vi "Initialize.vi"(7 "Channel Name":string="Setpoint.ch%d.SP", 8 "error in":errorcluster, 9 "Number of Channels":u32=1, 10 "Instance Name":string, 11 "Output Enable in":refnum<class "Output Enable.lvclass">) -> (0 "error out":errorcluster, 3 "Output Enable out":refnum<class "Output Enable.lvclass">)   [LabVIEW 2023, in "Output Enable.lvclass"]
uses:
  Output Enable.lvclass
  Output Enable.lvclass/Output Enable.ctl
  <vilib>/ADAS Replay HIL/Channels/Tag Wrapper/Tag Wrapper.lvlib
  Utilities/Utilities.lvlib
  <vilib>/ADAS Replay HIL/Channels/Tag Wrapper/Polymorphic/Set Default Value (Boolean).vi
  <vilib>/ADAS Replay HIL/Channels/Tag Wrapper/Polymorphic/Open Consumer Tag (Boolean).vi
  <vilib>/ADAS Replay HIL/Channels/Tag Wrapper/Polymorphic/Open Producer Tag (I32).vi
  <vilib>/ADAS Replay HIL/Channels/Tag Wrapper/Polymorphic/Set Default Value (I32).vi
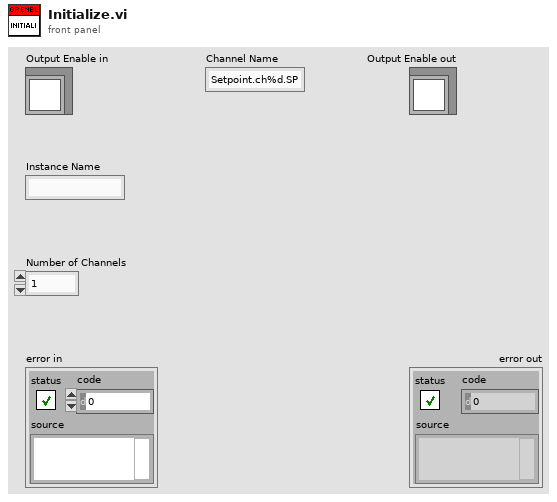
[diagram p1: front panel]
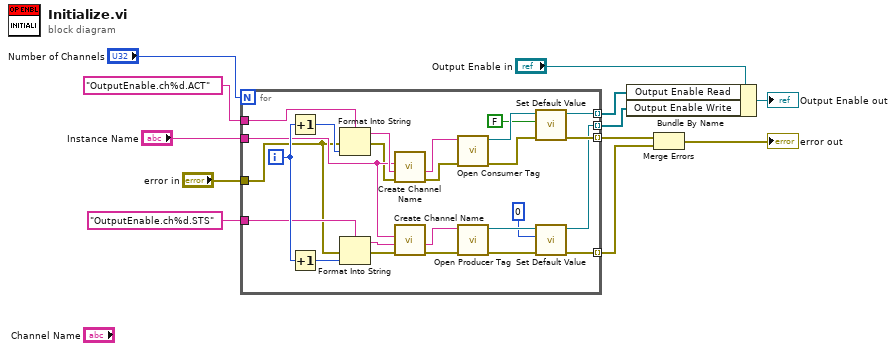
[diagram p0: block diagram]
diagram:
  n1 = for {
    N: "Number of Channels" -> [_]
    tunnel: "OutputEnable.ch%d.ACT" ("ChannelName") -> [w36]
    tunnel: "Instance Name" -> [w21]
    tunnel: "error in" -> [w14]
    tunnel: [w30] -> w7 mode=indexing
    tunnel: [w26] -> w6 mode=indexing
    tunnel: "OutputEnable.ch%d.STS" ("ChannelName") -> [w22]
    tunnel: [w19] -> w3 mode=indexing
    tunnel: [w18] -> w2 mode=indexing
    i -> [w23]
    n2 = Increment(x=w23) -> (x+1=w37:i32)
    n3 = Increment(x=w23) -> (x+1=w24:i32)
    n4 = Format Into String(format string=w36, error in=w14, w37) -> (resulting string=w35:string, error out=w16:errorcluster)  [unwired: 1 in]
    n5 = Format Into String(format string=w22, error in=w14, w24) -> (resulting string=w20:string, error out=w15:errorcluster)  [unwired: 1 in]
    n6 = call "Create Channel Name.vi"("error in"=w16, "Channel Name"=w35, "Plugin Name"=w21) -> ("error out"=w17:errorcluster, "Data Channel Name"=w34:string)  [unwired: 7 in]
    n7 = call "Create Channel Name.vi"("error in"=w15, "Channel Name"=w20, "Plugin Name"=w21) -> ("error out"=w28:errorcluster, "Data Channel Name"=w25:string)  [unwired: 7 in]
    n8 = call-poly <vilib>:"Open Consumer Tag.vi"("error in"=w17, "Channel Name"=w34) -> ("error out"=w32:errorcluster, "ADAS HIL Channel"=w33:refnum<k21>)  [unwired: 8 in]
    n9 = call-poly <vilib>:"Open Producer Tag.vi"("error in"=w28, "Channel Name"=w25) -> ("error out"=w27:errorcluster, "ADAS HIL Channel"=w29:refnum<k21>)  [unwired: 8 in]
    n10 = call-poly <vilib>:"Set Default Value.vi"("error in"=w32, "Default Value"=FALSE, "ADAS HIL Channel in"=w33) -> ("error out"=w30:errorcluster, "ADAS HIL Channel out"=w19:refnum<k21>)  [unwired: 7 in]
    n11 = call-poly <vilib>:"Set Default Value.vi"("error in"=w27, "Default Value"=0, "ADAS HIL Channel in"=w29) -> ("error out"=w26:errorcluster, "ADAS HIL Channel out"=w18:refnum<k21>)  [unwired: 7 in]
  }
  n12 = Bundle By Name(cluster="Output Enable in", "Output Enable Read"=w3, "Output Enable Write"=w2) -> (→"Output Enable out":refnum<class "Output Enable.lvclass">)
  n13 = Merge Errors(w7, w6) -> (→"error out":errorcluster)
